vi "test fpga pulse.vi"() -> ()   [LabVIEW 2015]
uses:
  <vilib>/Platform/TimedLoop/XDataNode/timing_clust.ctl
  <vilib>/Platform/TimedLoop/XDataNode/nitl_modes.ctl
  <vilib>/Platform/TimedLoop/XDataNode/wakeup.ctl
  <vilib>/rvi/Emulation/niFpgaSctlEmulationGetInTimedLoop.vi
  <vilib>/rvi/Emulation/niFpgaEmulationReportErrorSimple.vi
  <vilib>/rvi/Emulation/niFpgaGetClockAttributes.vi
  <vilib>/rvi/Emulation/niFpgaCriticalErrorInLSC.vi
  <vilib>/rvi/eio/common/nirviEmuTemplateMethod_errors.vi
  <vilib>/Platform/TimedLoop/XDataNode/XDataNode.xnode
  <vilib>/eio/EIONode/EIONode.xnode
  <vilib>/Platform/TimedLoop/XDataNode/XDNodeRunTimeDep.lvlib
  <instrlib>/_niInstr/Basic Elements/v1/FPGA/niInstr Basic Elements v1 FPGA.lvlib
panel:
  in  "Switch-1":bool
  in  "Pulse width":u32=200000 caption="计数器(滴答)"
  in  "FPGA Stop":bool
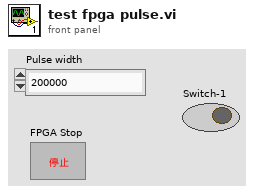
[diagram p1: front panel]
types:
  T1 = typedef "XDNodeRunTimeDep.lvlib/timing_clust.ctl" = cluster{"Expected End [f-1]":u64, "Actual End [f-1]":u64, "Finished Late? [f-1]":bool, "Expected End [i-1]":u64, "Actual End [i-1]":u64, "Finished Late? [i-1]":bool, "Expected Start [i]":u64, "Actual Start [i]":u64, "Expected Start [f]":u64, "Actual Start [f]":u64, "Source Name":string, "Structure Name":string, "Period":i64, "Deadline":i64, "Offset":i64, "Start":i64, "Priority":i32, "Timeout":i32, "Mode":T2, "Wakeup Reason":T3, "Error":errorcluster, "Source Type":string, "Secondary Source Type":string, "Global End Time":u64, "Global Start Time":u64, "Frame Duration":u64, "Iteration Duration":u64, "Assigned CPU":i32, "I/O Scan Engine Mode":u32}
  T2 = typedef "XDNodeRunTimeDep.lvlib/nitl_modes.ctl" = enum32{"No Change", "Process missed periods, maintain original phase", "Discard missed periods, maintain original phase", "Process missed periods, ignore original phase", "Discard missed periods, ignore original phase"}
  T3 = typedef "XDNodeRunTimeDep.lvlib/wakeup.ctl" = enum32{"Normal", "Aborted", "Asynchronous wakeup", "Timing source error", "Timed loop error", "Timeout"}
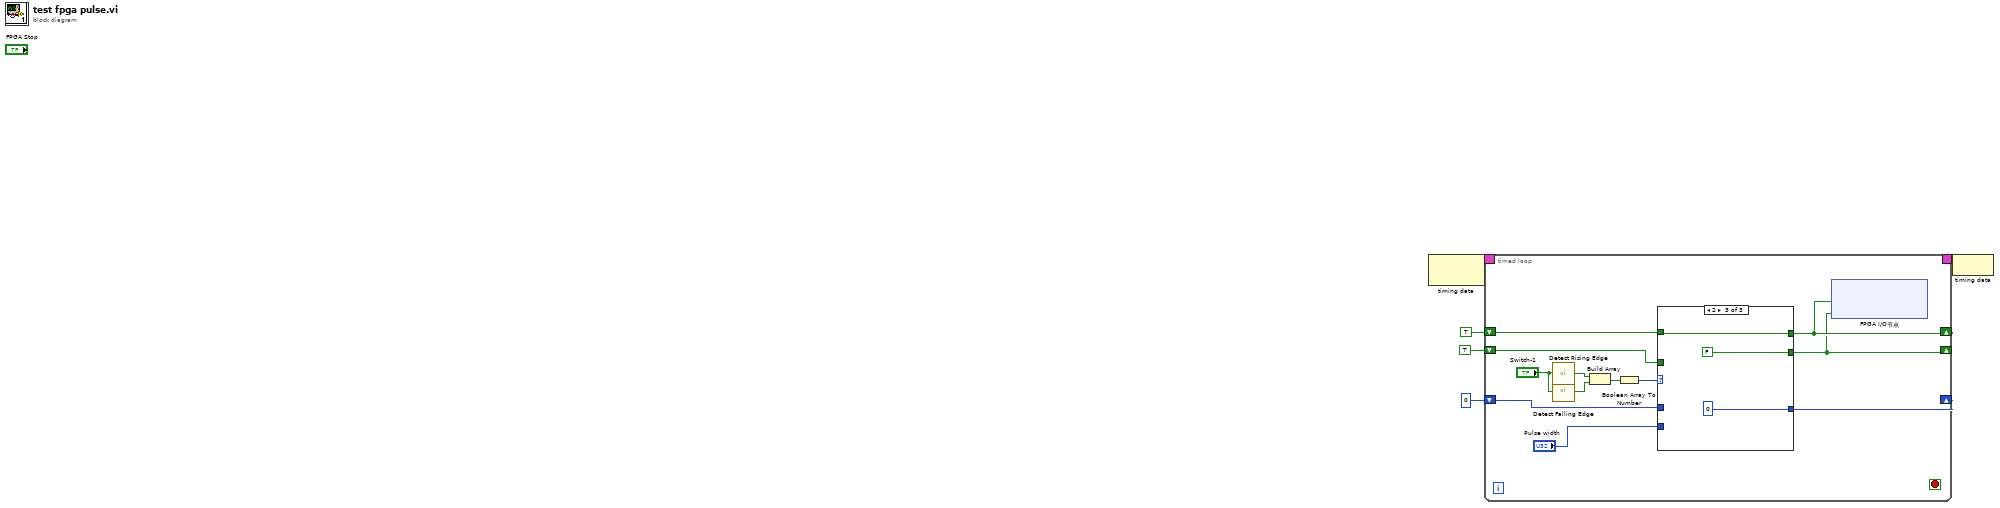
[diagram p0: block diagram]
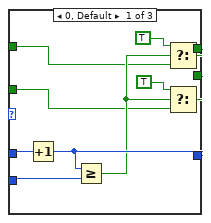
[diagram p2: hidden frame]
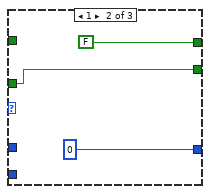
[diagram p3: hidden frame]
diagram:
  n1 = node-c288() -> (w5:T1)  [unwired: 1 in]
  n2 = timed-loop {
    shift-right: [w8] -> _
    shift-left: TRUE -> [w17]
    timing: w5 -> [_]
    timing-out: [_] -> w4
    shift-right: [w11] -> _
    shift-left: u32 0 ("MEMS FAST") -> [w16]
    shift-right: [w7] -> _
    shift-left: TRUE -> [w6]
    stop <- _ stop-if-true
    n3 = call <instrlib>:"Detect Rising Edge.vi"("signal"="Switch-1") -> ("edge detected"=w10:bool)  [unwired: 14 in]
    n4 = call <instrlib>:"Detect Falling Edge.vi"("signal"="Switch-1") -> ("edge detected"=w9:bool)  [unwired: 14 in]
    n5 = Build Array(w10, w9) -> (w13:bool[])
    n6 = Boolean Array To Number(Boolean array=w13) -> (number=w12:u8)
    n7 = case shown="2" w12 {
      tunnel: w17 -> [w20 _ w32]
      tunnel: w16 -> [w27 _ _]
      tunnel: "Pulse width" -> [w26 _ _]
      tunnel: [w25 u32 0 u32 0] -> w11
      tunnel: [w24 FALSE w32] -> w8
      tunnel: [w23 w29 FALSE ("f")] -> w7
      tunnel: w6 -> [w18 w29 _]
      frame 0, Default {
        n8 = Increment(x=w27) -> (x+1=w25:u32)
        n9 = Greater Or Equal?(x=w25, y=w26) -> (x >= y?=w22:bool)
        n10 = Select(t=TRUE ("f"), s=w22, f=w20) -> (s? t:f=w24:bool)
        n11 = Select(t=TRUE ("f"), s=w22, f=w18) -> (s? t:f=w23:bool)
      }
      frame 1 {
      }
      frame 2 {
      }
    }
    n12 = xnode "FPGA I/O节点"("Switch1.2/DIO6"=w8, "Switch-1.1/DIO7"=w7) -> ()  [unwired: 2 in, 2 out]
  }
  n13 = node-c288(w4) -> ()
